vi "PhaseCalcSubVI.vi"(0 "Phase Graph Reference":refnum<vi>, 1 "Wave_1":dbl[](array[numeric]), 2 "Wave_2":dbl[](array[numeric]), 3 "Error In":errorcluster, 4 "Number of Points/Period":i32) -> (6 "Phase":dbl, 7 "Error Out":errorcluster)   [LabVIEW 2022 SP3]
doc: "Inputs 2 waves in the form of 1 dimensional arrays and outputs the phase, a phase graph and an optional array of sum of difference values."
uses:
  <vilib>/Analysis/5stat.llb/RMS (DBL).vi
  <vilib>/Analysis/NI_AALPro.lvlib
panel:
  out "Phase Graph Out":cluster{dbl[], dbl[]}
  out "Sum of Difference Array":dbl[](array[numeric])
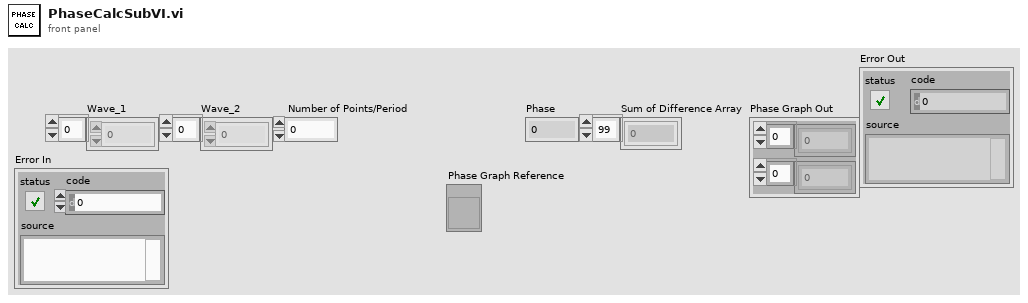
[diagram p1: front panel]
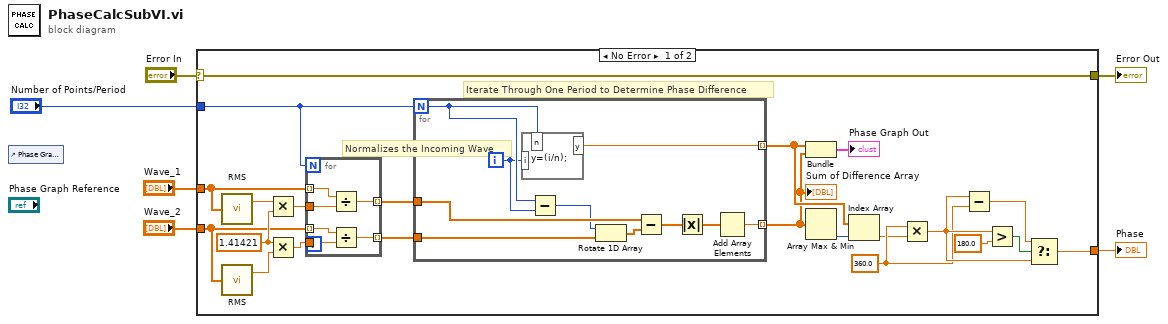
[diagram p0: block diagram]
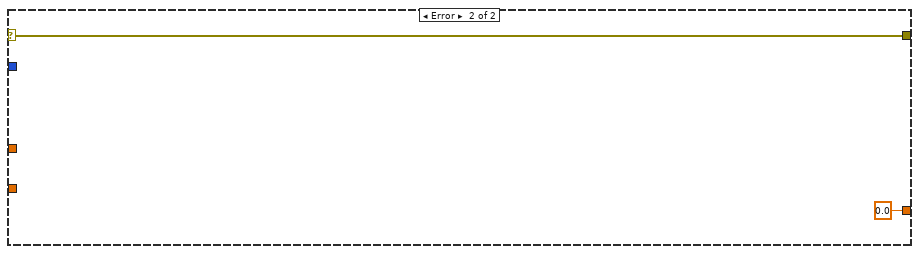
[diagram p2: hidden frame]
diagram:
  n1 = control-ref of="Phase Graph Out"() -> ()  [unwired: 1 out]
  n2 = case shown="No Error" "Error In" {
    selector: "Error In" -> [w7 w46]
    tunnel: [w28 0.0] -> w6
    tunnel: "Wave_2" -> [w11 _]
    tunnel: "Wave_1" -> [w10 _]
    tunnel: "Number of Points/Period" -> [w9 _]
    tunnel: [w7 w46] -> w2
    frame No Error {
      w16 = 1.41421
      w25 = 360.0 ("x")
      # "Normalizes the Incoming Wave"
      # "Iterate Through One Period to Determine Phase Difference"
      n3 = call-poly <vilib>:"RMS.vi"("X"=w10) -> ("rms value"=w14:dbl)  [unwired: 1 out]
      n4 = call-poly <vilib>:"RMS.vi"("X"=w11) -> ("rms value"=w15:dbl)  [unwired: 1 out]
      n5 = Multiply(x=w14, y=w16) -> (x*y=w13:dbl)
      n6 = Multiply(x=w16, y=w15) -> (x*y=w12:dbl)
      n7 = for {
        N: w9 -> [_]
        tunnel: [w34] -> w18 mode=indexing
        tunnel: [w33] -> w17 mode=indexing
        tunnel: w13 -> [w32]
        tunnel: w12 -> [w31]
        tunnel: w11 -> [w30] mode=indexing
        tunnel: w10 -> [w29] mode=indexing
        n8 = Divide(x=w29, y=w32) -> (x/y=w33:dbl)
        n9 = Divide(x=w30, y=w31) -> (x/y=w34:dbl)
      }
      n10 = for {
        N: w9 -> [w41]
        tunnel: w18 -> [w43]
        tunnel: w17 -> [w44]
        tunnel: [w35] -> w20 mode=indexing
        tunnel: [w36] -> w19 mode=indexing
        i -> [w39]
        n11 = formula code="y=(i/n);"("n"=w41, "i"=w39) -> ("y"=w35:dbl)
        n12 = Subtract(x=w41, y=w39) -> (x-y=w40:i32)
        n13 = Rotate 1D Array(1:w43, 2:w40) -> (0:w42:dbl[])
        n14 = Subtract(x=w44, y=w42) -> (x-y=w38:dbl[])
        n15 = Absolute Value(x=w38) -> (abs(x)=w37:dbl[])
        n16 = Add Array Elements(numeric array=w37) -> (sum=w36:dbl)
      }
      "Sum of Difference Array" <- w19
      n17 = Bundle(w20, w19) -> (→"Phase Graph Out":cluster{dbl[], dbl[]})  [unwired: 1 in]
      n18 = Array Max & Min(array=w19) -> (min index (indices)=w21:i32)  [unwired: 3 out]
      n19 = Index Array(array=w20, index=w21) -> (element=w22:dbl)
      n20 = Multiply(x=w25, y=w22) -> (x*y=w27:dbl)
      n21 = Subtract(x=w27, y=w25) -> (x-y=w26:dbl)
      n22 = Greater?(x=w27, y=180.0) -> (0:w24:bool)
      n23 = Select(t=w26, s=w24, f=w27) -> (s? t:f=w28:dbl)
    }
    frame Error {
    }
  }
  "Phase" <- w6
  "Error Out" <- w2
